vi "tmp.vi"() -> ()   [LabVIEW 2010]
panel:
  in  "Ch1":enum16{"Vin", "Vout", "Current", "Temp"}(ring)
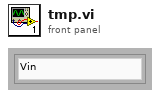
[diagram p1: front panel]
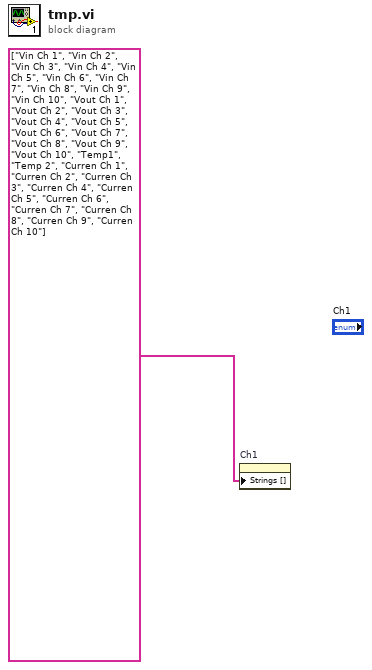
[diagram p0: block diagram]
diagram:
  n1 = property on="Ch1" class="Enum (strict)"("Strings []"=string[] ["Vin Ch 1", "Vin Ch 2", "Vin Ch 3", "Vin Ch 4", "Vin Ch 5", "Vin Ch 6", "Vin Ch 7", "Vin Ch 8", "Vin Ch 9", "Vin Ch 10", "Vout Ch 1", "Vout Ch 2", "Vout Ch 3", "Vout Ch 4", "Vout Ch 5", "Vout Ch 6", "Vout Ch 7", "Vout Ch 8", "Vout Ch 9", "Vout Ch 10", "Temp1", "Temp 2", "Curren Ch 1", "Curren Ch 2", "Curren Ch 3", "Curren Ch 4", "Curren Ch 5", "Curren Ch 6", "Curren Ch 7", "Curren Ch 8", "Curren Ch 9", "Curren Ch 10"]) -> ()  [unwired: 2 in, 2 out]
